vi "FPGA Set LED State.vi"(8 "error in (no error)":errorcluster, 9 "State":bool, 10 "LED":u8, 11 "Command":enum16{"Set LED", "Initialise"}(ring)) -> (0 "error out":errorcluster)   [LabVIEW 2017]
doc: "Updates the LED indicators on the MyRIO via FPGA front panel communication."
uses:
  FPGA Global Variables.vi
  <vilib>/Utility/error.llb/Error Cluster From Error Code.vi
  <vilib>/rvi/errors/niLvFpgaAdjustHostInterfaceError.vi
  <vilib>/rvi/interface/nirviReadWriteControl/nirviReadWriteControl.xnode
  NiFpgaLv.dll
  <vilib>/rvi/interface/Simulation/niFpgaSimulationCallBeginRW.vi
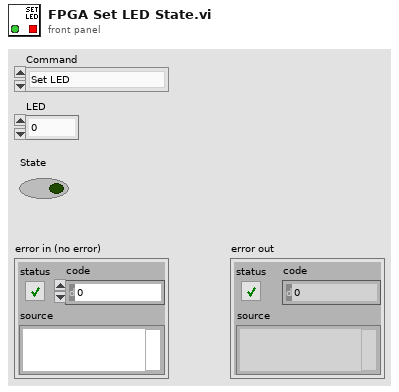
[diagram p1: front panel]
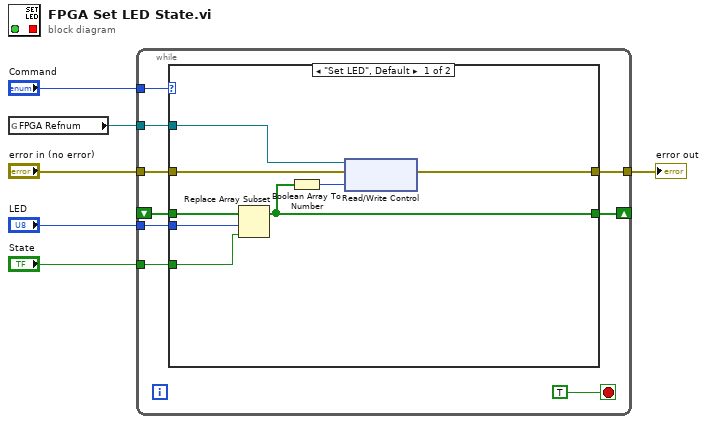
[diagram p0: block diagram]
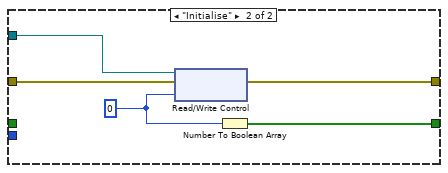
[diagram p2: hidden frame]
diagram:
  n1 = global read "FPGA Global Variables.vi" "FPGA Refnum"() -> (w5:refnum<k20>)
  n2 = while {
    tunnel: "Command" -> [w14]
    tunnel: w5 -> [w13]
    shift-right: [w12] -> _
    shift-left: _ -> [w11]
    tunnel: "LED" -> [w10]
    tunnel: "State" -> [w9]
    tunnel: "error in (no error)" -> [w8]
    tunnel: [w7] -> w1
    stop <- TRUE stop-if-true
    n3 = case shown="\"Set LED\", Default" w14 {
      tunnel: w13 -> [w23 w28]
      tunnel: [w16 w26] -> w12
      tunnel: w11 -> [w22 _]
      tunnel: w10 -> [w21 _]
      tunnel: w9 -> [w20 _]
      tunnel: w8 -> [w18 w24]
      tunnel: [w17 w25] -> w7
      frame "Set LED", Default {
        n4 = Replace Array Subset(array=w22, new element=w20, index=w21) -> (w16:bool[])
        n5 = Boolean Array To Number(Boolean array=w16) -> (number=w19:u8)
        n6 = xnode "Read/Write Control"("FPGA VI Reference In"=w23, "error in"=w18, "LED States"=w19) -> ("error out"=w17:errorcluster)  [unwired: 1 out]
      }
      frame "Initialise" {
        w27 = u8 0
        n7 = xnode "Read/Write Control"("FPGA VI Reference In"=w28, "error in"=w24, "LED States"=w27) -> ("error out"=w25:errorcluster)  [unwired: 1 out]
        n8 = Number To Boolean Array(number=w27) -> (Boolean array=w26:bool[])
      }
    }
  }
  "error out" <- w1
